vi "6_1_2.vi"() -> ()   [LabVIEW 2025, in "2022.lvlib"]
uses:
  2022.lvlib
panel:
  in  "6_1 / 6_2":bool
  out "Result":i32
  out "Array":string[](array[string])
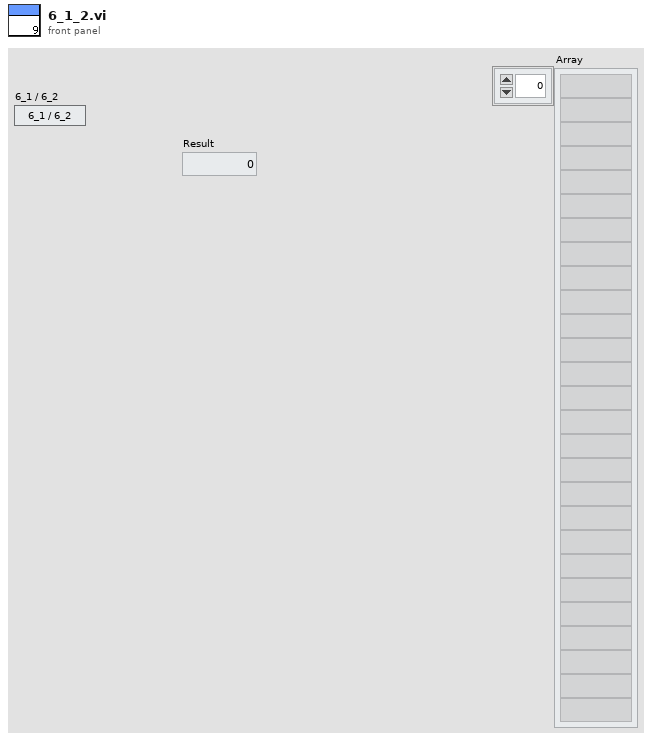
[diagram p1: front panel]
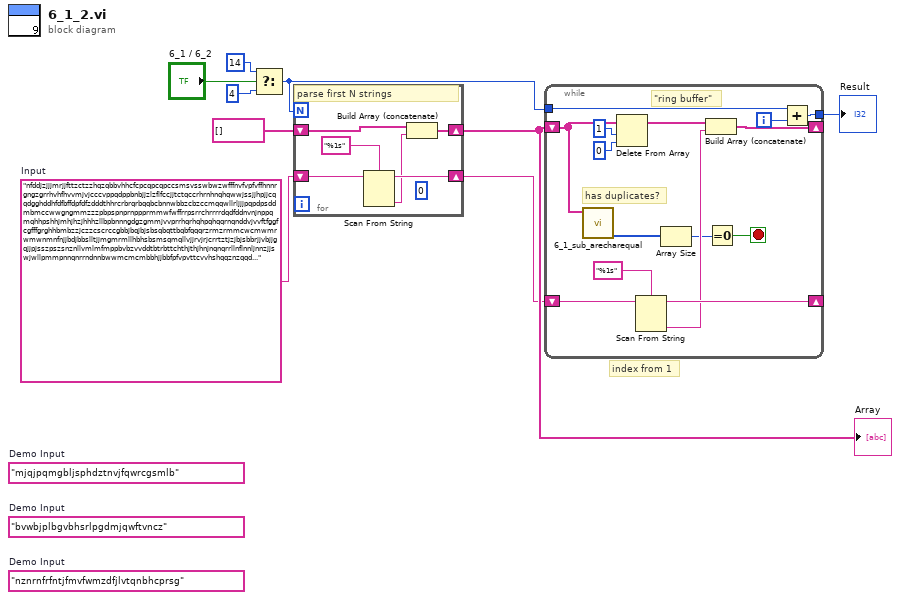
[diagram p0: block diagram]
diagram:
  (unwired) "nznrnfrfntjfmvfwmzdfjlvtqnbhcprsg"  # Demo Input
  (unwired) "bvwbjplbgvbhsrlpgdmjqwftvncz"  # Demo Input
  (unwired) "mjqjpqmgbljsphdztnvjfqwrcgsmlb"  # Demo Input
  w5 = "nfddjzjjjmrjjfttzctzzhqzqbbvhhcfcpcqpcqpccsmsvsswbwzwfffnvfvpfvffhnnrgngzgrrhvhfhvvmjvjcccvppqdppbnbjjzlzflfccjjtctqccrhrnhnqhqwwjssjjhpjjcqqdgghddhfdfbffdpfdfzdddthhrcrbrqrbqqbcbnnwbbzcbzccmqqwllrljjjpqpdpsddmbmccwwgngmmzzzpbpspnprnppprmmwfwffrrpsrrchrrrrdqdfddnvnjnppqmqhhpshhjmhjhzjhhhzllbpbnnngdgzgmmjvvprrhqrhqhpqhqqrnqnddvjvvftfggfcgfffgrghhbmbzzjczzcscrccgbbjbqjbjsbsqbqttbqbfqqqrzrmzrmmcwcmwmrwmwnmnfnjjbdjbbslltjjmgmrmllhbhsbsmsqmqllvjjrvjrjcrrtztjzjbjsbbrjjvbjjgqjjpjsszpszsnznllvmlmfmppbvbzvvddtbtrbttchthjthjhnjnqnqrrllnflnnljnnzjjswjwllpmmpnnqnrrndnnbwwmcmcmbbhjjbbfpfvpvttcvvhshqqznzqqd..."  # Input
  # "index from 1"
  n1 = Select(t=14, s="6_1 / 6_2", f=4) -> (s? t:f=w2:i32)
  n2 = for {
    N: w2 -> [_]
    shift-right: [w13] -> w7
    shift-left: w5 -> [w15]
    shift-right: [w10] -> w9
    shift-left: string[] [] -> [w12]
    (unwired) 0 ("index")
    # "parse first N strings"
    n3 = Scan From String(format string="%1s", input string=w15) -> (remaining string=w13:string, output 1=w11:string)  [unwired: 3 in, 2 out]
    n4 = Build Array (concatenate)(w12, w11) -> (w10:string[])
  }
  "Array" <- w9
  n5 = while {
    shift-right: [w20] -> _
    shift-left: w9 -> [w19]
    tunnel: w2 -> [w29]
    tunnel: [w28] -> w8
    shift-right: [w26] -> _
    shift-left: w7 -> [w27]
    i -> [w30]
    stop <- w16 stop-if-true
    # "\"ring buffer\""
    # "has duplicates?"
    n6 = call "6_1_sub_arecharequal.vi"("Array in"=w19) -> ("indices of removed elements"=w18:i32[])  [unwired: 10 in]
    n7 = Delete From Array(array=w19, length=1, index=0) -> (array with subset deleted=w22:string[])  [unwired: 1 out]
    n8 = Scan From String(format string="%1s", input string=w27) -> (remaining string=w26:string, output 1=w21:string)  [unwired: 3 in, 2 out]
    n9 = Array Size(array=w18) -> (size(s)=w17:i32)
    n10 = Build Array (concatenate)(w22, w21) -> (w20:string[])
    n11 = Equal To 0?(x=w17) -> (x = 0?=w16:bool)
    n12 = Add(x=w29, y=w30) -> (x+y=w28:i32)
  }
  "Result" <- w8
